vi "29.vi"() -> ()   [LabVIEW 2021]
panel:
  out "size":i32
  in  "b":i32
  in  "a":i32
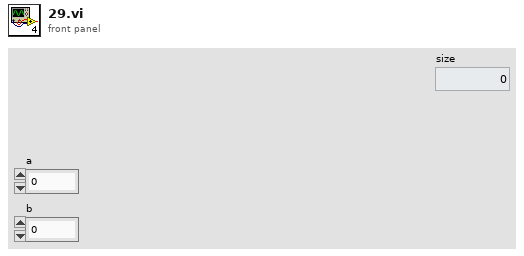
[diagram p1: front panel]
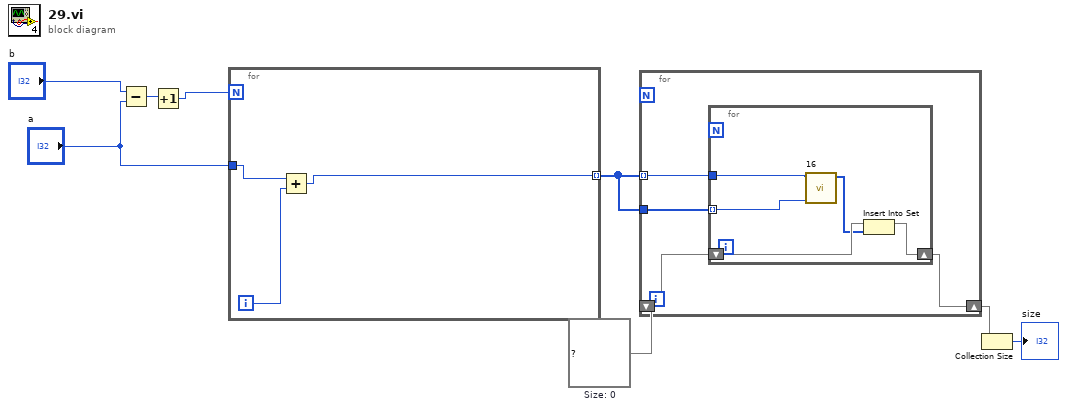
[diagram p0: block diagram]
diagram:
  w1 = set{u8[]} {}  # Size: 0
  n1 = Subtract(x="b", y="a") -> (x-y=w7:i32)
  n2 = Increment(x=w7) -> (x+1=w6:i32)
  n3 = for {
    N: w6 -> [_]
    tunnel: "a" -> [w11]
    tunnel: [w9] -> w4 mode=indexing
    i -> [w10]
    n4 = Add(x=w11, y=w10) -> (x+y=w9:i32)
  }
  n5 = for {
    tunnel: w4 -> [w15] mode=indexing
    tunnel: w4 -> [w14]
    shift-right: [w12] -> w3
    shift-left: w1 -> [w13]
    n6 = for {
      tunnel: w15 -> [w18]
      tunnel: w14 -> [w17] mode=indexing
      shift-right: [w19] -> w12
      shift-left: w13 -> [w20]
      n7 = call "16.vi"("base"=w17, "exponent"=w18) -> ("reversed array 2"=w16:u8[])  [unwired: 9 in]
      n8 = Insert Into Set(10:w16, 11:w20) -> (3:w19:set{u8[]})  [unwired: 1 out]
    }
  }
  n9 = Collection Size(1:w3) -> (0:→"size":i32)
